vi "变长数组.vi"() -> ()   [LabVIEW 2012]
panel:
  out "变长数组":cluster{"CH0":dbl[], "CH1":dbl[], "CH2":dbl[]}[](array[cluster])
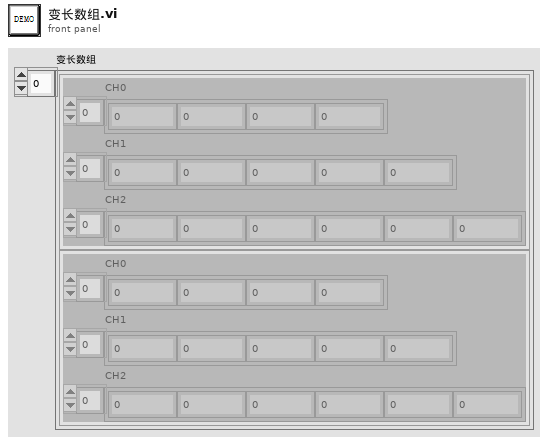
[diagram p1: front panel]
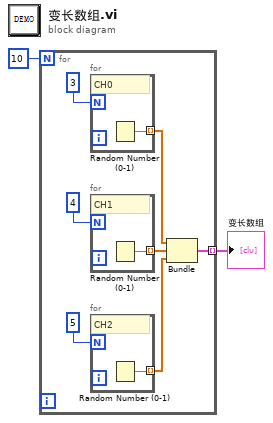
[diagram p0: block diagram]
diagram:
  n1 = for {
    N: 10 -> [_]
    tunnel: [w3] -> w1 mode=indexing
    n2 = for {
      N: 3 -> [_]
      tunnel: [w12] -> w6 mode=indexing
      # "CH0"
      n3 = Random Number (0-1)() -> (number: 0 to 1=w12:dbl)
    }
    n4 = for {
      N: 4 -> [_]
      tunnel: [w11] -> w5 mode=indexing
      # "CH1"
      n5 = Random Number (0-1)() -> (number: 0 to 1=w11:dbl)
    }
    n6 = for {
      N: 5 -> [_]
      tunnel: [w10] -> w4 mode=indexing
      # "CH2"
      n7 = Random Number (0-1)() -> (number: 0 to 1=w10:dbl)
    }
    n8 = Bundle(w6, w5, w4) -> (w3:cluster{dbl[], dbl[], dbl[]})  [unwired: 1 in]
  }
  "变长数组" <- w1
